vi "FlatToRichGreeter_res.vi"(5 "OutputClusterType":T1, 11 "InputCluster":T2) -> (3 "OutputCluster":T1)   [LabVIEW 2019, in "Generated_server.lvlib"]
uses:
  Generated_server.lvlib
  Greeter_res_Flat.ctl
  Greeter_res.ctl
  Greeter_res_res_oneof/Greeter_res_res_oneof.lvclass
  Greeter_res_res_oneof/Greeter_res_res_oneof.lvclass/Greeter_res_res_oneof.ctl
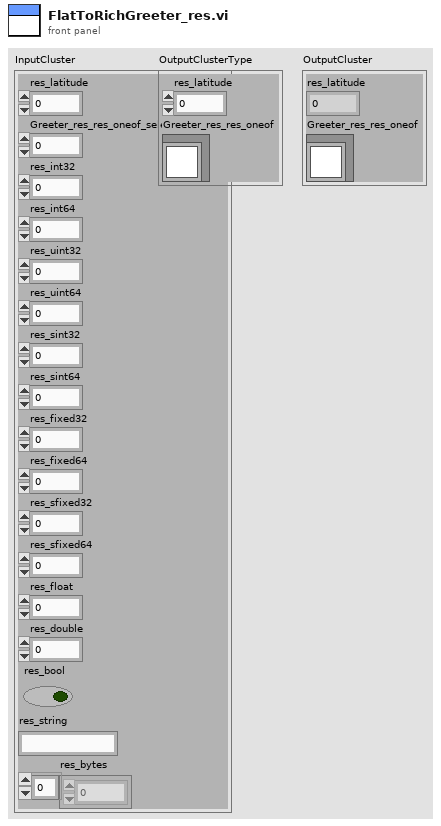
[diagram p1: front panel]
types:
  T1 = typedef "Generated_server.lvlib/Greeter_res.ctl" = cluster{"res_latitude":i32, "Greeter_res_res_oneof":refnum<class "Greeter_res_res_oneof.lvclass">}
  T2 = typedef "Generated_server.lvlib/Greeter_res_Flat.ctl" = cluster{"res_latitude":i32, "Greeter_res_res_oneof_selected_index":i32, "res_int32":i32, "res_int64":i64, "res_uint32":u32, "res_uint64":u64, "res_sint32":i32, "res_sint64":i64, "res_fixed32":u32, "res_fixed64":u64, "res_sfixed32":i32, "res_sfixed64":i64, "res_float":sgl, "res_double":dbl, "res_bool":bool, "res_string":string, "res_bytes":u8[]}
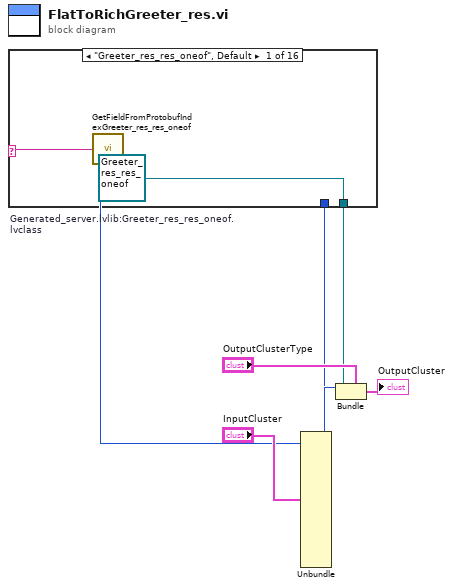
[diagram p0: block diagram]
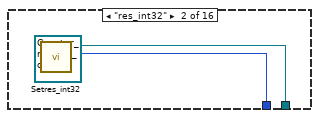
[diagram p2: hidden frame]
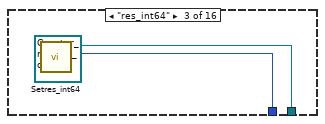
[diagram p3: hidden frame]
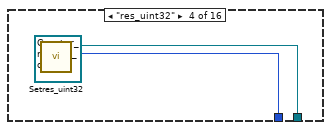
[diagram p4: hidden frame]
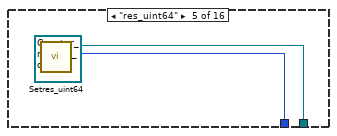
[diagram p5: hidden frame]
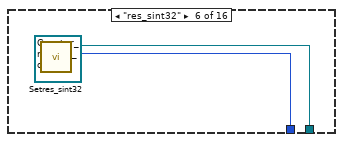
[diagram p6: hidden frame]
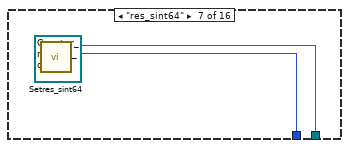
[diagram p7: hidden frame]
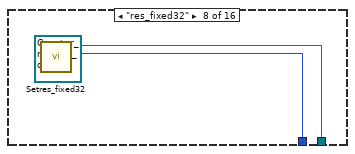
[diagram p8: hidden frame]
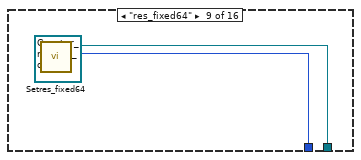
[diagram p9: hidden frame]
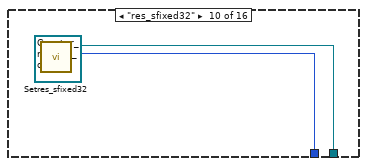
[diagram p10: hidden frame]
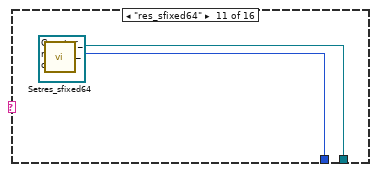
[diagram p11: hidden frame]
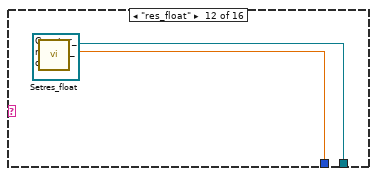
[diagram p12: hidden frame]
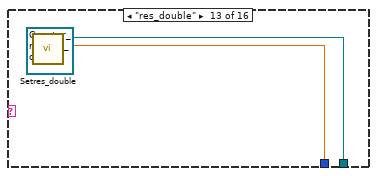
[diagram p13: hidden frame]
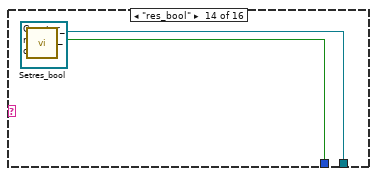
[diagram p14: hidden frame]
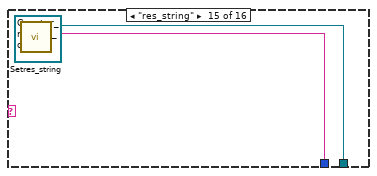
[diagram p15: hidden frame]
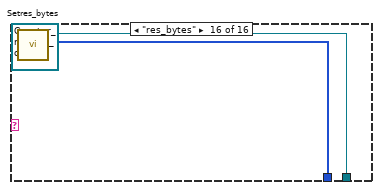
[diagram p16: hidden frame]
diagram:
  n1 = Unbundle "Unbundle"("InputCluster") -> ("res_latitude"=w19:i32, "Greeter_res_res_oneof_selected_index"=w18:i32, "res_int32"=w15:i32, "res_int64"=w14:i64, "res_uint32"=w13:u32, "res_uint64"=w12:u64, "res_sint32"=w11:i32, "res_sint64"=w10:i64, "res_fixed32"=w9:u32, "res_fixed64"=w8:u64, "res_sfixed32"=w7:i32, "res_sfixed64"=w6:i64, "res_float"=w5:sgl, "res_double"=w4:dbl, "res_bool"=w3:bool, "res_string"=w2:string, "res_bytes"=w1:u8[])
  n2 = call "GetFieldFromProtobufIndexGreeter_res_res_oneof.vi"("protobuf index"=w18) -> ("oneof field name"=w17:string)
  n3 = case "Greeter_res_res_oneof" shown="\"Greeter_res_res_oneof\", Default" w17 {
    tunnel: [w23 w25 w28 w31 w34 w37 w40 w43 w46 w49 w52 w55 w58 w61 w64 w67] -> w16
    tunnel: w15 -> [_ w26 _ _ _ _ _ _ _ _ _ _ _ _ _ _]
    tunnel: w14 -> [_ _ w29 _ _ _ _ _ _ _ _ _ _ _ _ _]
    tunnel: w13 -> [_ _ _ w32 _ _ _ _ _ _ _ _ _ _ _ _]
    tunnel: w12 -> [_ _ _ _ w35 _ _ _ _ _ _ _ _ _ _ _]
    tunnel: w11 -> [_ _ _ _ _ w38 _ _ _ _ _ _ _ _ _ _]
    tunnel: w10 -> [_ _ _ _ _ _ w41 _ _ _ _ _ _ _ _ _]
    tunnel: w9 -> [_ _ _ _ _ _ _ w44 _ _ _ _ _ _ _ _]
    tunnel: w8 -> [_ _ _ _ _ _ _ _ w47 _ _ _ _ _ _ _]
    tunnel: w7 -> [_ _ _ _ _ _ _ _ _ w50 _ _ _ _ _ _]
    tunnel: w6 -> [_ _ _ _ _ _ _ _ _ _ w53 _ _ _ _ _]
    tunnel: w5 -> [_ _ _ _ _ _ _ _ _ _ _ w56 _ _ _ _]
    tunnel: w4 -> [_ _ _ _ _ _ _ _ _ _ _ _ w59 _ _ _]
    tunnel: w3 -> [_ _ _ _ _ _ _ _ _ _ _ _ _ w62 _ _]
    tunnel: w2 -> [_ _ _ _ _ _ _ _ _ _ _ _ _ _ w65 _]
    tunnel: w1 -> [_ _ _ _ _ _ _ _ _ _ _ _ _ _ _ w68]
    frame "Greeter_res_res_oneof", Default {
      w23 = refnum<class "Greeter_res_res_oneof.lvclass"> refnum  # Generated_server.lvlib:Greeter_res_res_oneof.lvclass
    }
    frame "res_int32" {
      n4 = call "Setres_int32.vi"("Set_Val"=w26, "OneOfTemplate in"=refnum<class "Greeter_res_res_oneof.lvclass"> refnum) -> ("OneOfTemplate out"=w25:refnum<class "Greeter_res_res_oneof.lvclass">)  [unwired: 8 in, 1 out]
    }
    frame "res_int64" {
      n5 = call "Setres_int64.vi"("Set_Val"=w29, "OneOfTemplate in"=refnum<class "Greeter_res_res_oneof.lvclass"> refnum) -> ("OneOfTemplate out"=w28:refnum<class "Greeter_res_res_oneof.lvclass">)  [unwired: 8 in, 1 out]
    }
    frame "res_uint32" {
      n6 = call "Setres_uint32.vi"("Set_Val"=w32, "OneOfTemplate in"=refnum<class "Greeter_res_res_oneof.lvclass"> refnum) -> ("OneOfTemplate out"=w31:refnum<class "Greeter_res_res_oneof.lvclass">)  [unwired: 8 in, 1 out]
    }
    frame "res_uint64" {
      n7 = call "Setres_uint64.vi"("Set_Val"=w35, "OneOfTemplate in"=refnum<class "Greeter_res_res_oneof.lvclass"> refnum) -> ("OneOfTemplate out"=w34:refnum<class "Greeter_res_res_oneof.lvclass">)  [unwired: 8 in, 1 out]
    }
    frame "res_sint32" {
      n8 = call "Setres_sint32.vi"("Set_Val"=w38, "OneOfTemplate in"=refnum<class "Greeter_res_res_oneof.lvclass"> refnum) -> ("OneOfTemplate out"=w37:refnum<class "Greeter_res_res_oneof.lvclass">)  [unwired: 8 in, 1 out]
    }
    frame "res_sint64" {
      n9 = call "Setres_sint64.vi"("Set_Val"=w41, "OneOfTemplate in"=refnum<class "Greeter_res_res_oneof.lvclass"> refnum) -> ("OneOfTemplate out"=w40:refnum<class "Greeter_res_res_oneof.lvclass">)  [unwired: 8 in, 1 out]
    }
    frame "res_fixed32" {
      n10 = call "Setres_fixed32.vi"("Set_Val"=w44, "OneOfTemplate in"=refnum<class "Greeter_res_res_oneof.lvclass"> refnum) -> ("OneOfTemplate out"=w43:refnum<class "Greeter_res_res_oneof.lvclass">)  [unwired: 8 in, 1 out]
    }
    frame "res_fixed64" {
      n11 = call "Setres_fixed64.vi"("Set_Val"=w47, "OneOfTemplate in"=refnum<class "Greeter_res_res_oneof.lvclass"> refnum) -> ("OneOfTemplate out"=w46:refnum<class "Greeter_res_res_oneof.lvclass">)  [unwired: 8 in, 1 out]
    }
    frame "res_sfixed32" {
      n12 = call "Setres_sfixed32.vi"("Set_Val"=w50, "OneOfTemplate in"=refnum<class "Greeter_res_res_oneof.lvclass"> refnum) -> ("OneOfTemplate out"=w49:refnum<class "Greeter_res_res_oneof.lvclass">)  [unwired: 8 in, 1 out]
    }
    frame "res_sfixed64" {
      n13 = call "Setres_sfixed64.vi"("Set_Val"=w53, "OneOfTemplate in"=refnum<class "Greeter_res_res_oneof.lvclass"> refnum) -> ("OneOfTemplate out"=w52:refnum<class "Greeter_res_res_oneof.lvclass">)  [unwired: 8 in, 1 out]
    }
    frame "res_float" {
      n14 = call "Setres_float.vi"("Set_Val"=w56, "OneOfTemplate in"=refnum<class "Greeter_res_res_oneof.lvclass"> refnum) -> ("OneOfTemplate out"=w55:refnum<class "Greeter_res_res_oneof.lvclass">)  [unwired: 8 in, 1 out]
    }
    frame "res_double" {
      n15 = call "Setres_double.vi"("Set_Val"=w59, "OneOfTemplate in"=refnum<class "Greeter_res_res_oneof.lvclass"> refnum) -> ("OneOfTemplate out"=w58:refnum<class "Greeter_res_res_oneof.lvclass">)  [unwired: 8 in, 1 out]
    }
    frame "res_bool" {
      n16 = call "Setres_bool.vi"("Set_Val"=w62, "OneOfTemplate in"=refnum<class "Greeter_res_res_oneof.lvclass"> refnum) -> ("OneOfTemplate out"=w61:refnum<class "Greeter_res_res_oneof.lvclass">)  [unwired: 8 in, 1 out]
    }
    frame "res_string" {
      n17 = call "Setres_string.vi"("Set_Val"=w65, "OneOfTemplate in"=refnum<class "Greeter_res_res_oneof.lvclass"> refnum) -> ("OneOfTemplate out"=w64:refnum<class "Greeter_res_res_oneof.lvclass">)  [unwired: 8 in, 1 out]
    }
    frame "res_bytes" {
      n18 = call "Setres_bytes.vi"("Set_Val"=w68, "OneOfTemplate in"=refnum<class "Greeter_res_res_oneof.lvclass"> refnum) -> ("OneOfTemplate out"=w67:refnum<class "Greeter_res_res_oneof.lvclass">)  [unwired: 8 in, 1 out]
    }
  }
  n19 = Bundle "Bundle"(cluster="OutputClusterType", "res_latitude"=w19, "Greeter_res_res_oneof"=w16) -> (→"OutputCluster":T1)
